vi "PH_IEEE1394Camera.search Cam.vi"(0 "i ref in":refnum<vi>, 2 "Cam ID (Serial Number)":string, 4 "Cam Error in":errorcluster) -> (15 "Available Cams":string[](array[string]), 16 "Cam found":bool, 17 "Cam.Name (machinery)":string, 18 "Cam Error out":errorcluster)   [LabVIEW 2014, in "PH_IEEE1394Camera.lvlib"]
doc: "This VI searches out of all connected cams the wanted: It gives out the \"Cam.Name (machinery)\" if one of the cams\n\n1) has the same name as the instance, or\n2) has the same name as the \"Cam Info\", or\n3) has the same hexidecimal seral number as the \"Cam Info\", or\n4) has the same serial number as as the \"Cam Info\".\n\nOtherwise \"N/A\" is indicated."
uses:
  PH_IEEE1394Camera.lvlib
  <vilib>/vision/driver/NI_Vision_Acquisition_Software.lvlib
  CSCore/CSSystem/CSSystemLib/CSSystemLib.lvlib
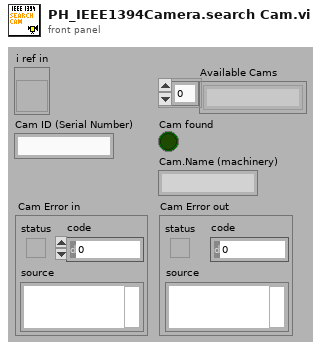
[diagram p1: front panel]
types:
  T1 = cluster{"Type":u32, "Version":u32, "Flags":u32, "SerialNumberHigh":u32, "SerialNumberLow":u32, "BusType":u32, "InterfaceName":string, "VendorName":string, "ModelName":string, "CameraFileName":string, "CameraAttributeURL":string}[]
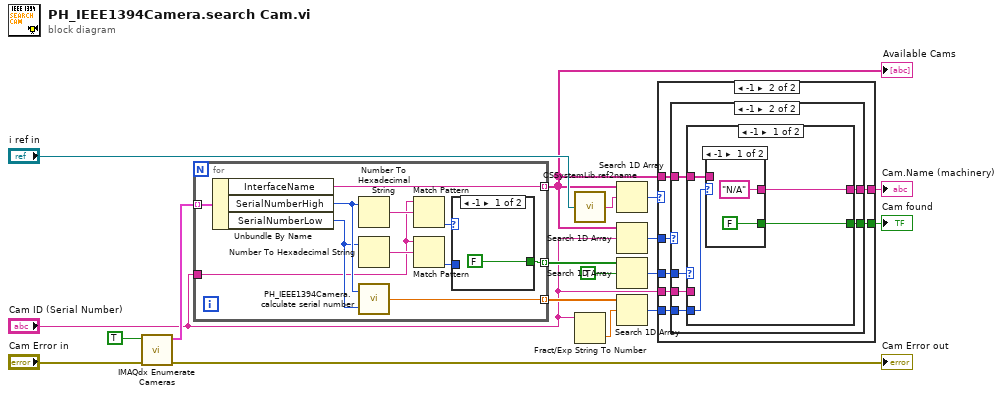
[diagram p0: block diagram]
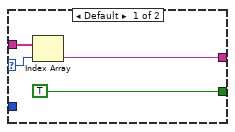
[diagram p2: hidden frame]
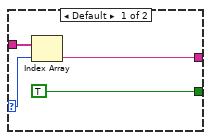
[diagram p3: hidden frame]
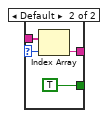
[diagram p4: hidden frame]
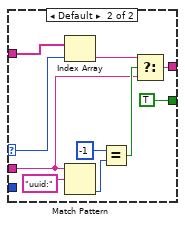
[diagram p5: hidden frame]
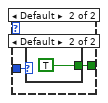
[diagram p6: hidden frame]
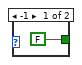
[diagram p7: hidden frame]
diagram:
  n1 = call <vilib>:"IMAQdx Enumerate Cameras.vi"("error in"="Cam Error in", "Connected Only? (Yes)"=TRUE) -> ("error out"=→"Cam Error out":errorcluster, "Camera Information Array"=w18:T1)  [unwired: 8 in]
  n2 = for {
    tunnel: w18 -> [w29] mode=indexing
    tunnel: [w20] -> w10 mode=indexing
    tunnel: [w28] -> w6 mode=indexing
    tunnel: "Cam ID (Serial Number)" -> [w23]
    tunnel: [w19] -> w8 mode=indexing
    n3 = Unbundle By Name(w29) -> ("InterfaceName"=w20:string, "SerialNumberHigh"=w26:u32, "SerialNumberLow"=w25:u32)
    n4 = Number To Hexadecimal String(2:w26) -> (0:w27:string)  [unwired: 1 in]
    n5 = Number To Hexadecimal String(2:w25) -> (0:w24:string)  [unwired: 1 in]
    n6 = call "PH_IEEE1394Camera.calculate serial number.vi"("SerialNumberLow"=w25, "SerialNumberHigh"=w26) -> ("Serial Number"=w28:dbl)
    n7 = Match Pattern(string=w23, regular expression=w27) -> (offset past match=w22:i32)  [unwired: 1 in, 3 out]
    n8 = Match Pattern(string=w23, regular expression=w24) -> (offset past match=w21:i32)  [unwired: 1 in, 3 out]
    n9 = case shown="-1" w22 {
      tunnel: w21 -> [_ w32]
      tunnel: [FALSE w31] -> w19
      frame -1 {
      }
      frame Default {
        n10 = case shown="Default" w32 {
          tunnel: [FALSE TRUE] -> w31
          frame -1 {
          }
          frame Default {
          }
        }
      }
    }
  }
  "Available Cams" <- w10
  n11 = call "CSSystemLib.ref2name.vi"("obj refnum"="i ref in") -> ("name"=w13:string)
  n12 = Fract/Exp String To Number(string="Cam ID (Serial Number)") -> (number=w4:dbl)  [unwired: 3 in, 1 out]
  n13 = Search 1D Array(1D array=w10, element=w13) -> (index of element=w12:i32)  [unwired: 1 in]
  n14 = Search 1D Array(1D array=w10, element="Cam ID (Serial Number)") -> (index of element=w11:i32)  [unwired: 1 in]
  n15 = Search 1D Array(1D array=w8, element=TRUE) -> (index of element=w7:i32)  [unwired: 1 in]
  n16 = Search 1D Array(1D array=w6, element=w4) -> (index of element=w5:i32)  [unwired: 1 in]
  n17 = case shown="-1" w12 {
    selector: w12 -> [w37 _]
    tunnel: [w36 w45] -> w17
    tunnel: w10 -> [w38 w44]
    tunnel: w11 -> [_ w43]
    tunnel: w7 -> [_ w42]
    tunnel: w5 -> [_ w41]
    tunnel: [TRUE w40] -> w3
    tunnel: "Cam ID (Serial Number)" -> [_ w39]
    frame Default {
      n18 = Index Array(array=w38, index=w37) -> (element=w36:string)
    }
    frame -1 {
      n19 = case shown="-1" w43 {
        selector: w43 -> [w47 _]
        tunnel: w44 -> [w49 w55]
        tunnel: [w48 w54] -> w45
        tunnel: w42 -> [_ w53]
        tunnel: w41 -> [_ w52]
        tunnel: [TRUE w51] -> w40
        tunnel: w39 -> [_ w50]
        frame Default {
          n20 = Index Array(array=w49, index=w47) -> (element=w48:string)
        }
        frame -1 {
          n21 = case shown="-1" w53 {
            selector: w53 -> [_ w67]
            tunnel: w55 -> [w59 w68]
            tunnel: [w58 w69] -> w54
            tunnel: w52 -> [w57 _]
            tunnel: [w56 TRUE] -> w51
            tunnel: w50 -> [_ w70]
            frame -1 {
              n22 = case shown="-1" w57 {
                selector: w57 -> [_ w63]
                tunnel: w59 -> [_ w65]
                tunnel: ["N/A" ("InterfaceName") w64] -> w58
                tunnel: [FALSE TRUE] -> w56
                frame -1 {
                }
                frame Default {
                  n23 = Index Array(array=w65, index=w63) -> (element=w64:string)
                }
              }
            }
            frame Default {
              n24 = Index Array(array=w68, index=w67) -> (element=w66:string)
              n25 = Match Pattern(string=w70, regular expression="uuid:") -> (offset past match=w73:i32)  [unwired: 1 in, 3 out]
              n26 = Equal?(x=-1, y=w73) -> (x = y?=w71:bool)
              n27 = Select(t=w66, s=w71, f=w70) -> (s? t:f=w69:string)
            }
          }
        }
      }
    }
  }
  "Cam.Name (machinery)" <- w17
  "Cam found" <- w3
